vi "hse-application_GetApplicationInfos.vi"(8 "error in":errorcluster) -> (0 "error out":errorcluster, 1 "Application Name":string, 2 "Application Unit-ID":string, 3 "Application Title":string)   [LabVIEW 2020, in "hse-application.lvclass"]
doc: "Returns information on the application itself for display, logging, ...\n\n\n\n____\nHAMPEL SOFTWARE ENGINEERING v3.8.0 (2023-12-18 14:41)"
uses:
  hse-application.lvclass
  hse-application.lvclass/hse-application.ctl
  <vilib>/Utility/error.llb/Error Cluster From Error Code.vi
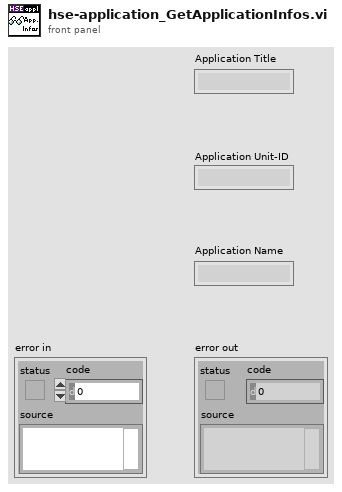
[diagram p1: front panel]
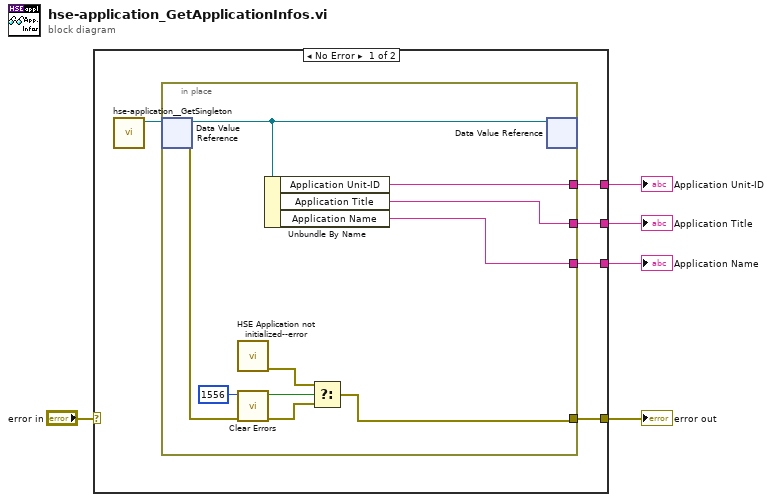
[diagram p0: block diagram]
diagram:
  n1 = case shown="No Error" "error in" {
    selector: "error in" -> [_ w21]
    tunnel: [w10 w21] -> w4
    tunnel: [w8 _] -> w3
    tunnel: [w7 _] -> w2
    tunnel: [w6 _] -> w1
    frame No Error {
      n2 = call "hse-application__GetSingleton.vi"() -> ("ApplicationClass DVR"=w9:refnum<data-value>)  [unwired: 10 in, 1 out]
      n3 = in-place {
        in-place-border: [w17] -> w10
        in-place-border: [w15] -> w8
        in-place-border: [w14] -> w7
        in-place-border: [w13] -> w6
        n4 = in-place-dvr #1(w9) -> (w16:refnum<class "hse-application.lvclass">, w20:errorcluster)
        n5 = call "HSE Application not initialized--error.vi"() -> ("error out"=w19:errorcluster)  [unwired: 11 in]
        n6 = call <vilib>:"Clear Errors.vi"("error in (no error)"=w20, "specific error code to clear (0: all)"=1556) -> ("error out"=w18:errorcluster, "specific error cleared?"=w11:bool)  [unwired: 4 in]
        n7 = Unbundle By Name(w16) -> ("Application Unit-ID"=w14:string, "Application Title"=w15:string, "Application Name"=w13:string)
        n8 = Select(t=w19, s=w11, f=w18) -> (s? t:f=w17:errorcluster)
        n9 = in-place-dvr #1(w16) -> ()  [unwired: 2 out]
      }
    }
    frame Error {
    }
  }
  "error out" <- w4
  "Application Title" <- w3
  "Application Unit-ID" <- w2
  "Application Name" <- w1
